vi "生产者消费者.vi"() -> ()   [LabVIEW 2015]
doc: "该模板用于创建生产者／消费者模式的应用程序，以事件驱动的方式，生成队列中的项。如需通过响应事件实现代码的异步执行，同时不影响用户界面的响应速度，可考虑用该模式替代用户界面事件处理器模式。"
panel:
  in  "Enqueue Element":bool caption="元素入队列"
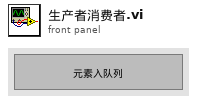
[diagram p1: front panel]
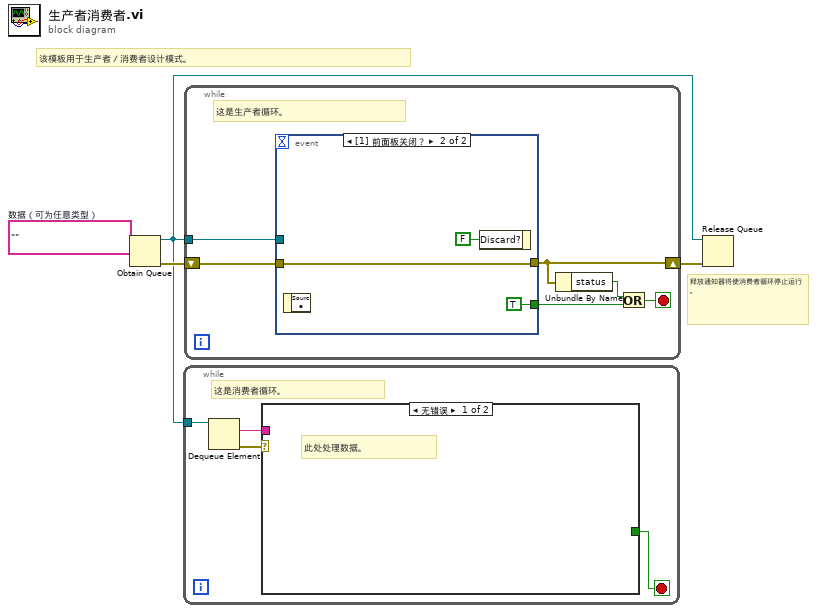
[diagram p0: block diagram]
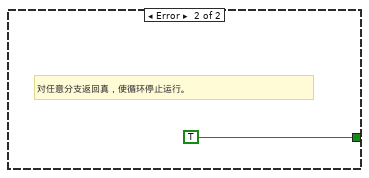
[diagram p2: hidden frame]
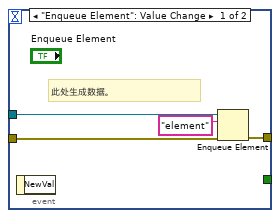
[diagram p3: hidden frame]
diagram:
  w2 = ""  # 数据（可为任意类型）
  # "释放通知器将使消费者循环停止运行。"
  # "该模板用于生产者／消费者设计模式。"
  n1 = Obtain Queue(element data type=w2) -> (queue out=w1:refnum<queue>, error out=w4:errorcluster)  [unwired: 4 in, 1 out]
  n2 = while {
    tunnel: w1 -> [w8]
    stop <- w5 stop-if-true
    # "这是消费者循环。"
    n3 = Dequeue Element(queue=w8) -> (element=w6:string, error out=w7:errorcluster)  [unwired: 2 in, 2 out]
    n4 = case shown="无错误" w7 {
      tunnel: w6 -> [_ _]
      tunnel: [_ TRUE] -> w5
      frame No Error {
        # "此处处理数据。"
      }
      frame Error {
        # "对任意分支返回真，使循环停止运行。"
      }
    }
  }
  n5 = while {
    shift-right: [w11] -> w3
    shift-left: w4 -> [w14]
    tunnel: w1 -> [w15]
    stop <- w12 stop-if-true
    # "这是生产者循环。"
    n6 = event shown="[1] 前面板关闭？" {
      selector: _ -> [_ _]
      dyn-events: _ -> [_ _]
      timeout: _ -> [_ _]
      tunnel: w15 -> [w19 _]
      tunnel: w14 -> [w18 w22]
      tunnel: [w17 w22] -> w11
      tunnel: [_ TRUE ("stop")] -> w13
      event "Enqueue Element": Value Change {
        # "此处生成数据。"
        n7 = event-data() -> ()  [unwired: 1 in, 1 out]
        n8 = Enqueue Element(queue=w19, element="element", error in (no error)=w18) -> (error out=w17:errorcluster)  [unwired: 1 in, 2 out]
      }
      event Panel Close? {
        n9 = event-data() -> ()  [unwired: 1 in, 1 out]
        n10 = event-data("Discard?"=FALSE ("放弃？")) -> ()  [unwired: 1 in, 1 out]
      }
    }
    n11 = Unbundle By Name(w11) -> ("status"=w10:bool)
    n12 = Or(x=w10, y=w13) -> (x .or. y?=w12:bool)
  }
  n13 = Release Queue(queue=w1, error in (no error)=w3) -> ()  [unwired: 1 in, 3 out]
